vi "Tipo de señal.vi"(8 "error in (no error)":errorcluster, 10 "Tipo de señal":u16(ring), 11 "Generador funciones in":refnum<class "Generador funciones.lvclass">) -> (0 "error out":errorcluster, 3 "Generador funciones out":refnum<class "Generador funciones.lvclass">)   [LabVIEW 2019, in "Generador funciones.lvlib" / "Generador funciones.lvclass"]
uses:
  Generador funciones.lvclass
  Generador funciones.lvclass/Generador funciones.ctl
  <vilib>/ActorFramework/Message Enqueuer/Message Enqueuer.lvclass/Message Enqueuer.ctl
  <vilib>/ActorFramework/Message Enqueuer/Enqueue.vi
  C:/Program Files/National Instruments/LabVIEW 2019/vi.lib/ActorFramework/Message/Message.lvclass
  <vilib>/ActorFramework/Message Priority Queue/Priority Enqueue.vi
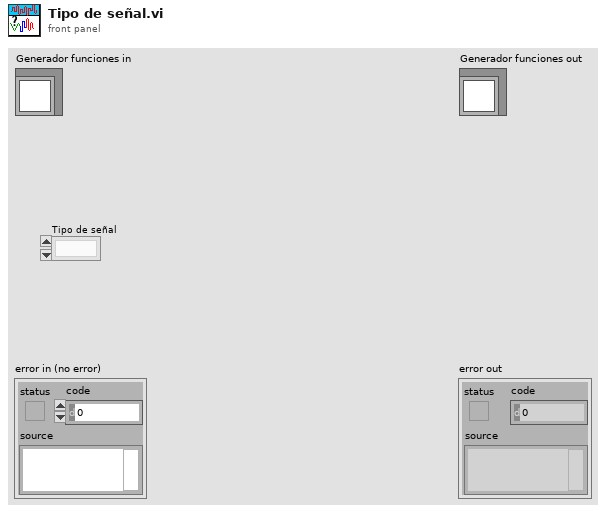
[diagram p1: front panel]
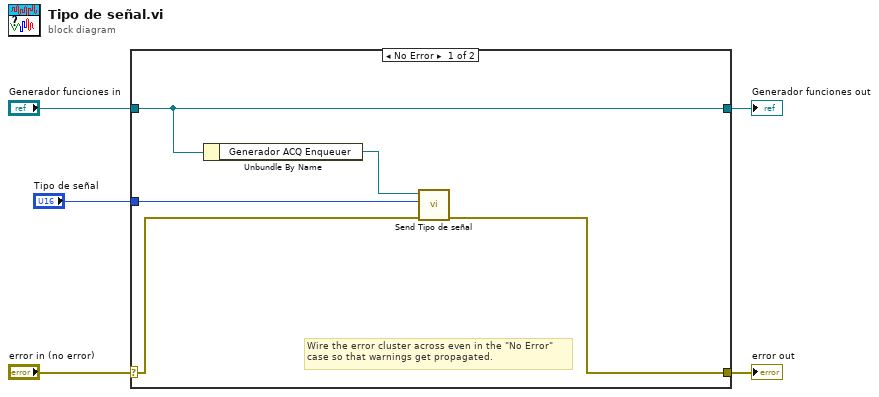
[diagram p0: block diagram]
diagram:
  n1 = case shown="No Error" "error in (no error)" {
    selector: "error in (no error)" -> [w7 w12]
    tunnel: [w6 w12] -> w4
    tunnel: [w10 w11] -> w2
    tunnel: "Generador funciones in" -> [w10 w11]
    tunnel: "Tipo de señal" -> [w8 _]
    frame No Error {
      # "Wire the error cluster across even in the \"No Error\"\ncase so that warnings get propagated."
      n2 = Unbundle By Name(w10) -> ("Generador ACQ Enqueuer"=w9:refnum<class "Message Enqueuer.lvclass">)
      n3 = call "Send Tipo de señal.vi"("error in (no error)"=w7, "Tipo de señal"=w8, "Message Enqueuer"=w9) -> ("error out"=w6:errorcluster)  [unwired: 7 in, 1 out]
    }
    frame Error {
    }
  }
  "error out" <- w4
  "Generador funciones out" <- w2
